vi "CSV_Change_to_SI_Notation.vi"(11 "CSV File Path":path=path "D:/Ngene/GitHub/culab_examples/Benchmarks/CuLab_Simple_Benchmarks/LabVIEW/Results/Intel(R) Core(TM) i7-8700K___NVIDIA GeForce RTX 2080 Ti/Conv1D_Top.csv") -> (3 "new file path":path)   [LabVIEW 2020]
uses:
  <vilib>/Utility/file.llb/Write Delimited Spreadsheet (string).vi
  <vilib>/Utility/file.llb/Read Delimited Spreadsheet (string).vi
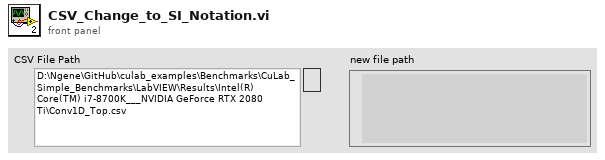
[diagram p1: front panel]
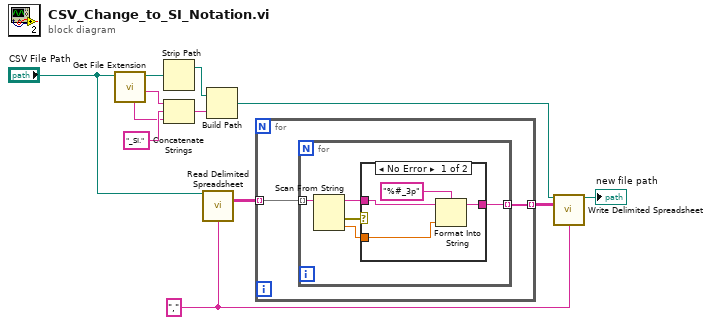
[diagram p0: block diagram]
diagram:
  w1 = "," ("delimiter (\\t)")
  n1 = call <vilib>:"Get File Extension.vi"("file"="CSV File Path") -> ("filename without extension"=w9:string, "dup file"=w6:path, "unmodified file extension"=w7:string)  [unwired: 6 in, 2 out]
  n2 = Strip Path(path=w6) -> (stripped path=w5:path)  [unwired: 1 out]
  n3 = Concatenate Strings(w9, "_SI." ("string"), w7) -> (w4:string)
  n4 = call-poly <vilib>:"Read Delimited Spreadsheet.vi"("file path (dialog if empty)"="CSV File Path", "delimiter (\\t)"=w1) -> ("all rows"=w12:string[][])  [unwired: 8 in, 5 out]
  n5 = Build Path(base path=w5, name or relative path=w4) -> (appended path=w3:path)
  n6 = for {
    tunnel: w12 -> [w14] mode=indexing
    tunnel: [w13] -> w11 mode=indexing
    n7 = for {
      tunnel: w14 -> [w19] mode=indexing
      tunnel: [w15] -> w13 mode=indexing
      n8 = Scan From String(input string=w19) -> (remaining string=w17:string, error out=w18:errorcluster, output 1=w16:dbl)  [unwired: 4 in, 1 out]
      n9 = case shown="No Error" w18 {
        tunnel: w17 -> [w22 w24]
        tunnel: w16 -> [w23 _]
        tunnel: [w21 w24] -> w15
        frame No Error {
          n10 = Format Into String(format string="%#_3p", initial string=w22, w23) -> (resulting string=w21:string)  [unwired: 1 in, 1 out]
        }
        frame Error {
        }
      }
    }
  }
  n11 = call-poly <vilib>:"Write Delimited Spreadsheet.vi"("file path (dialog if empty)"=w3, "2D data"=w11, "delimiter (\\t)"=w1) -> ("new file path (Not A Path if cancelled)"=→"new file path":path)  [unwired: 11 in, 1 out]
